vi "Get_Table.vi"(0 "Sorted_Array":string[](array[string]), 11 "Error_In":errorcluster) -> (4 "Table":string[][](array[string]), 15 "Error_Out":errorcluster)   [LabVIEW 2023]
doc: "This VI gets the sorted array and build 2D array with S No and Size"
uses:
  Library/Custom_Sort_Library.lvlib
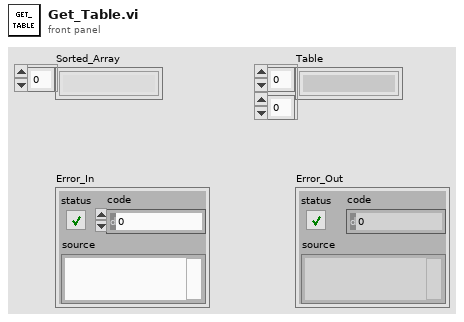
[diagram p1: front panel]
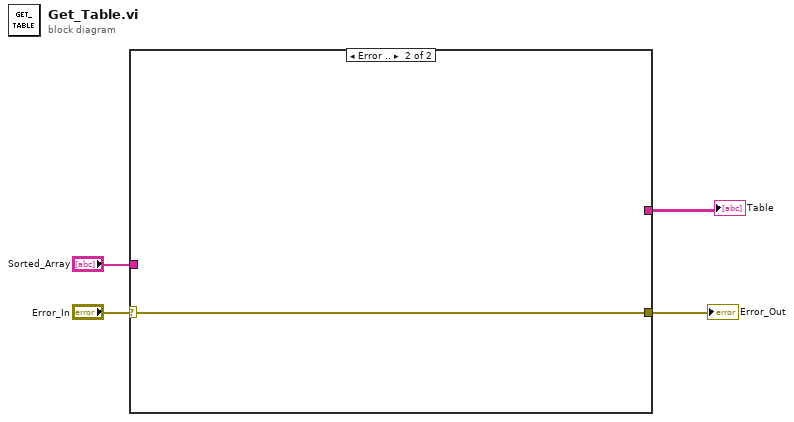
[diagram p0: block diagram]
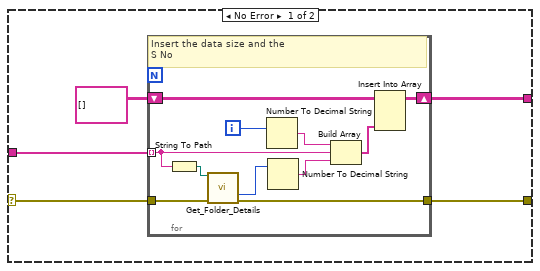
[diagram p2: hidden frame]
diagram:
  n1 = case shown="Error .." "Error_In" {
    selector: "Error_In" -> [w5 w21]
    tunnel: [w9 w21] -> w4
    tunnel: [w7 _] -> w3
    tunnel: "Sorted_Array" -> [w6 _]
    frame No Error {
      n2 = for {
        tunnel: w6 -> [w13] mode=indexing
        shift-right: [w16] -> w7
        shift-left: string[][] [] -> [w15]
        tunnel: w5 -> [w11]
        tunnel: [w10] -> w9
        i -> [w20]
        # "Insert the data size and the \nS No"
        n3 = String To Path(string=w13) -> (path=w14:path)
        n4 = call "Get_Folder_Details.vi"("Path"=w14, "Error_In"=w11) -> ("Size"=w12:i64, "Error_Out"=w10:errorcluster)  [unwired: 8 in, 4 out]
        n5 = Number To Decimal String(number=w20) -> (decimal integer string=w19:string)  [unwired: 1 in]
        n6 = Number To Decimal String(number=w12) -> (decimal integer string=w18:string)  [unwired: 1 in]
        n7 = Build Array(w19, w13, w18) -> (w17:string[])
        n8 = Insert Into Array(array=w15, new element=w17) -> (w16:string[][])  [unwired: 2 in]
      }
    }
    frame Error {
    }
  }
  "Error_Out" <- w4
  "Table" <- w3
